vi "SeCrTs-Enqueue Error_R.vi"(9 "error to process":errorcluster, 10 "Error Type (Non-Critical)":T1, 11 "Message Queue":refnum<queue>) -> ()   [LabVIEW 2022 SP3]
uses:
  RT Controls/Message Cluster_R.ctl
  RT Controls/Error Type_R.ctl
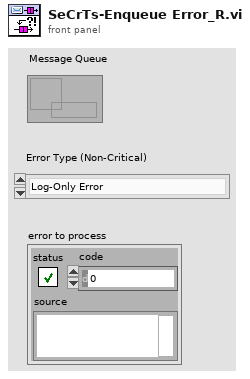
[diagram p1: front panel]
types:
  T1 = typedef "Error Type_R.ctl" = enum16{"Log-Only Error", "Non-Critical Error", "Critical Error"}
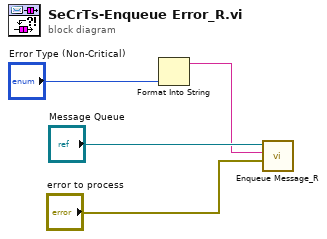
[diagram p0: block diagram]
diagram:
  n1 = Format Into String("Error Type (Non-Critical)") -> (resulting string=w2:string)  [unwired: 3 in, 1 out]
  n2 = call "Enqueue Message_R.vi"("Message Data"="error to process", "Message"=w2, "Message Queue"="Message Queue") -> ()  [unwired: 7 in, 2 out]
